vi "Util - Get All IP Addresses.vi"() -> (2 "Available IPs":string[](array[string]))   [LabVIEW 2019, in "UDP-Custom-Device Engine.lvlib"]
uses:
  UDP-Custom-Device Engine.lvlib
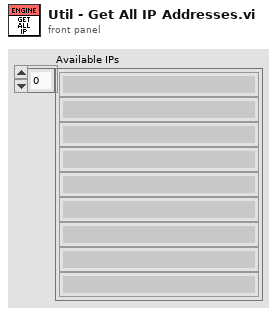
[diagram p1: front panel]
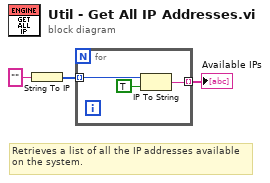
[diagram p0: block diagram]
diagram:
  # "Retrieves a list of all the IP addresses available\non the system."
  n1 = String To IP(1:"" ("name")) -> (0:w2:u32[])
  n2 = for {
    tunnel: w2 -> [w6] mode=indexing
    tunnel: [w4] -> w1 mode=indexing
    n3 = IP To String(1:TRUE ("dot notation? (F)"), 2:w6) -> (0:w4:string)
  }
  "Available IPs" <- w1
